vi "ROSTerminal.vi"() -> ()   [LabVIEW 2015]
doc: "Provides a space to debug any errors in code by:\n-allowing for testing connection to master\n-showing open nodes\n-linking to a website for viewing what is passed back and forth on a topic\n-linking to a website for the master to view what is passed back and forth\n-showing open logs\n-providing IP for you and Master"
uses:
  _ROSDefinition.vi
  vi.lib/Platform/browser.llb/Open URL in Default Browser (string).vi
  SubVIs/_ROSDirection.ctl
  SubVIs/_ROSControl.ctl
panel:
  in  "Change IP":bool
  in  "CloseServer":bool
  out "Queue Contents":string[](array[string])
  in  "ClearAllLogs":bool
  in  "CloseServers":bool
  in  "LabVIEW Servers":i32(listbox)
  in  "ClearOldLogs":bool
  in  "Web Logs":i32(listbox)
  in  "OpenNodes":bool
  in  "MasterWeb":bool
  in  "MyWeb":bool
  in  "UDP":bool
  out "My IP":string="http://192.168.1.8"
  in  "Done":bool
  out "Live":bool
  in  "Test":bool
  in  "Current Master":string="192.168.1.110:11311"
  # "Displays queue size and contents. Double click for\nmore information on a particular server."
  # "Show commands sent over TCP. \nDouble click to open a web page."
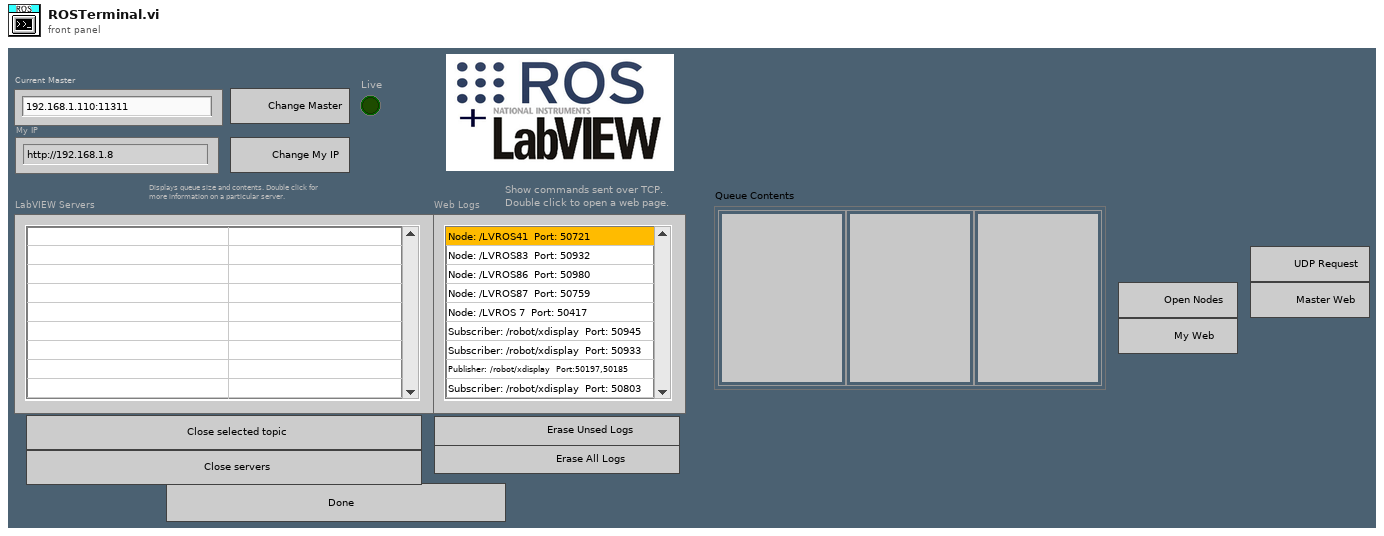
[diagram p1: front panel]
types:
  T1 = enum8{"Enabled", "Disabled", "Disabled and Grayed Out"}
  T2 = typedef "_ROSControl.ctl" = cluster{"topic port":u16, "Node":string, "topic":string, "type":string, "node port":u16, "error ":errorcluster, "Direction":T3, "Update (ms)":u16, "FIFO size":u16}
  T3 = typedef "_ROSDirection.ctl" = enum16{"Node", "Publisher", "Subscriber", "ServiceClient", "ServiceProvider"}
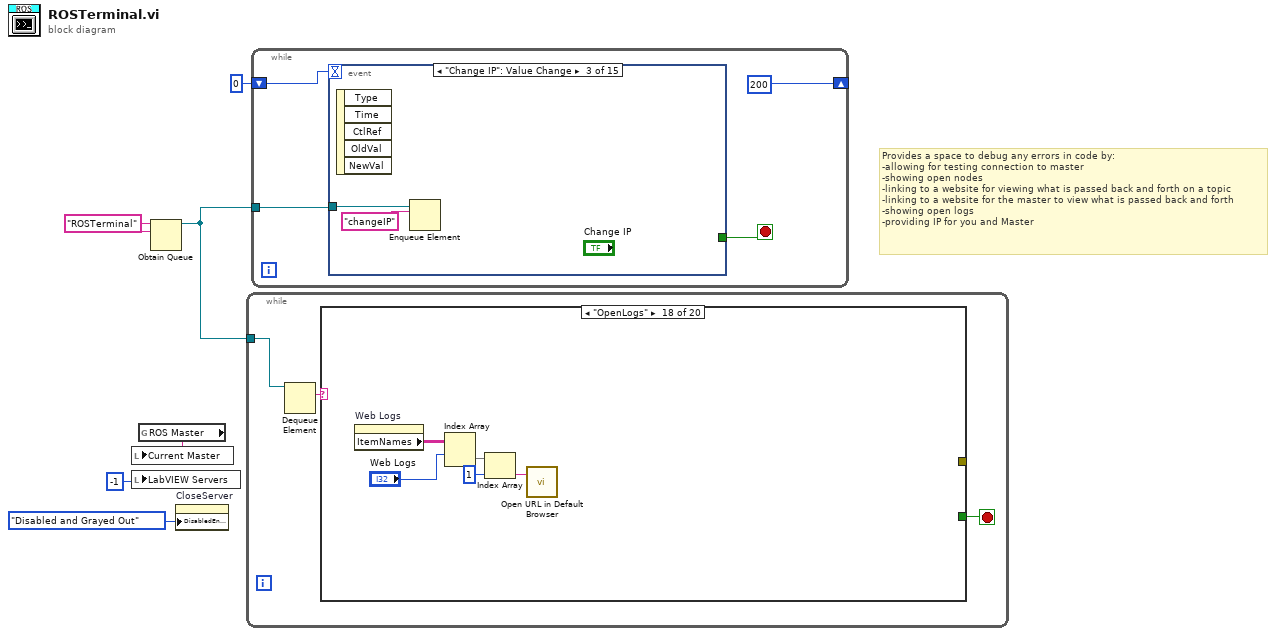
[diagram p0: block diagram]
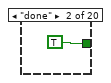
[diagram p3: hidden frame]
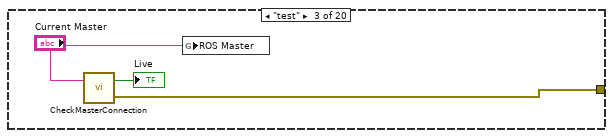
[diagram p4: hidden frame]
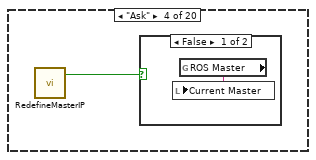
[diagram p5: hidden frame]
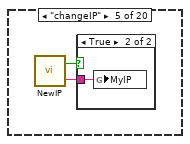
[diagram p7: hidden frame]
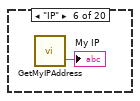
[diagram p9: hidden frame]
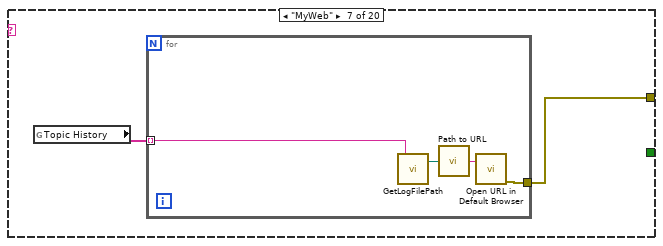
[diagram p10: hidden frame]
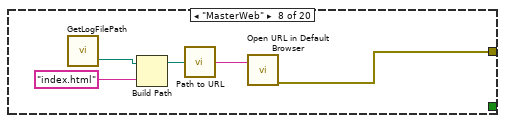
[diagram p11: hidden frame]
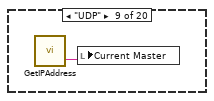
[diagram p12: hidden frame]
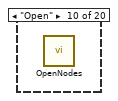
[diagram p13: hidden frame]
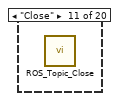
[diagram p14: hidden frame]
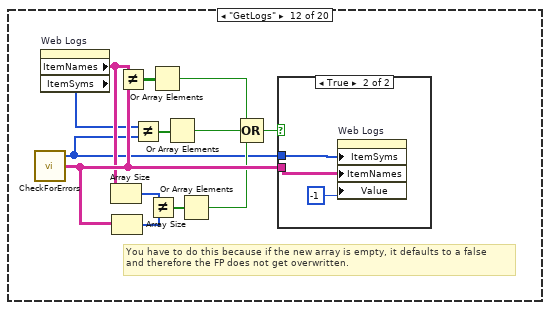
[diagram p15: hidden frame]
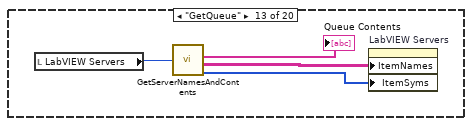
[diagram p17: hidden frame]
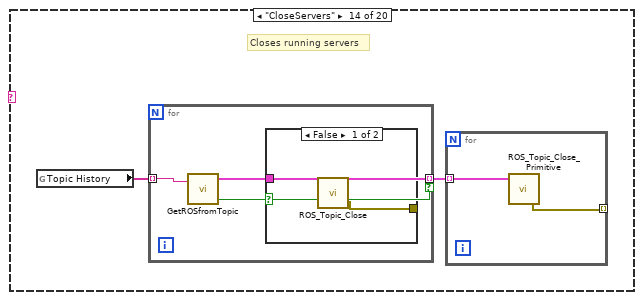
[diagram p18: hidden frame]
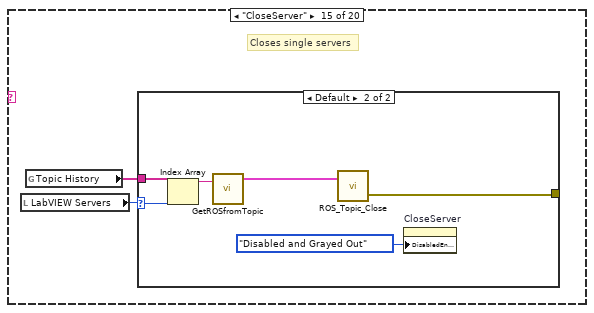
[diagram p20: hidden frame]
diagram:
  w5 = "ROSTerminal" ("name (unnamed)")
  # "Provides a space to debug any errors in code by:\n-allowing for testing connection to master\n-showing open nodes\n-linking to a website for viewing what is passed back and forth on a topic\n-linking to a website for the master to view what is passed back and forth\n-showing open logs\n-providing IP for you and Master"
  n1 = local write "LabVIEW Servers"(-1 ("Nodes")) -> ()
  n2 = global read "_ROSDefinition.vi" "ROS Master"() -> (w6:string)
  n3 = local write "Current Master"(w6) -> ()
  n4 = Obtain Queue(name (unnamed)=w5, element data type=w5) -> (queue out=w3:refnum<queue>)  [unwired: 3 in, 2 out]
  n5 = property on="CloseServer" class="Bool"("DisabledEnum"=T1."Disabled and Grayed Out" ("Disabled")) -> ()  [unwired: 2 in, 2 out]
  n6 = while {
    tunnel: w3 -> [w9]
    stop <- w7 stop-if-true
    n7 = Dequeue Element(queue=w9) -> (element=w8:string)  [unwired: 2 in, 3 out]
    n8 = case shown="\"OpenLogs\"" w8 {
      tunnel: [_ TRUE _ _ _ _ _ _ _ _ _ _ _ _ _ _ _ _ _ _] -> w7
      tunnel: [_ _ w11 _ _ _ w21 w26 _ _ _ _ _ _ _ w70 _ _ _ _] -> _
      frame Default {
      }
      frame "done" {
      }
      frame "test" {
        n9 = call "CheckMasterConnection.vi"("Master IP"="Current Master") -> ("error out"=w11:errorcluster, "Master There?"=→"Live":bool)  [unwired: 1 in]
        n10 = global write "_ROSDefinition.vi" "ROS Master"("Current Master") -> ()
      }
      frame "Ask" {
        n11 = call "RedefineMasterIP.vi"() -> ("Abort?"=w14:bool)  [unwired: 2 in]
        n12 = case shown="False" w14 {
          frame False {
            n13 = global read "_ROSDefinition.vi" "ROS Master"() -> (w15:string)
            n14 = local write "Current Master"(w15) -> ()
          }
          frame True {
          }
        }
      }
      frame "changeIP" {
        n15 = call "NewIP.vi"() -> ("New IP"=w16:string, "New IP?"=w17:bool)  [unwired: 2 in]
        n16 = case shown="True" w17 {
          tunnel: w16 -> [_ w18]
          frame False {
          }
          frame True {
            n17 = global write "_ROSDefinition.vi" "MyIP"(w18) -> ()
          }
        }
      }
      frame "IP" {
        n18 = call "GetMyIPAddress.vi"() -> ("URI"=→"My IP":string)  [unwired: 2 in, 1 out]
      }
      frame "MyWeb" {
        n19 = global read "_ROSDefinition.vi" "Topic History"() -> (w20:string[])
        n20 = for {
          tunnel: [w24] -> w21
          tunnel: w20 -> [w22] mode=indexing
          n21 = call "GetLogFilePath.vi"("Server name"=w22) -> ("LogPath"=w23:path)  [unwired: 1 in, 1 out]
          n22 = call "Path to URL.vi"("path"=w23) -> ("url"=w25:string)
          n23 = call-poly "Open URL in Default Browser.vi"("URL"=w25) -> ("error out"=w24:errorcluster)  [unwired: 5 in, 1 out]
        }
      }
      frame "MasterWeb" {
        n24 = call "GetLogFilePath.vi"() -> ("LogFolder"=w29:path)  [unwired: 2 in, 1 out]
        n25 = Build Path(base path=w29, name or relative path="index.html") -> (appended path=w27:path)
        n26 = call "Path to URL.vi"("path"=w27) -> ("url"=w30:string)
        n27 = call-poly "Open URL in Default Browser.vi"("URL"=w30) -> ("error out"=w26:errorcluster)  [unwired: 5 in, 1 out]
      }
      frame "UDP" {
        n28 = call "GetIPAddress.vi"() -> ("data out"=w31:string)  [unwired: 3 in]
        n29 = local write "Current Master"(w31) -> ()
      }
      frame "Open" {
        n30 = call "OpenNodes.vi"() -> ()  [unwired: 2 in]
      }
      frame "Close" {
        n31 = call "ROS_Topic_Close.vi"() -> ()  [unwired: 4 in, 1 out]
      }
      frame "GetLogs" {
        # "You have to do this because if the new array is empty, it defaults to a false\nand therefore the FP does not get overwritten."
        n32 = call "CheckForErrors.vi"() -> ("Symbols"=w33:i32[], "Logs"=w43:string[][])  [unwired: 2 in, 1 out]
        n33 = property on="Web Logs" class="MCListbox (strict)"() -> ("ItemNames"=w42:string[][], "ItemSyms"=w34:i32[])  [unwired: 2 in, 2 out]
        n34 = Array Size(array=w42) -> (size(s)=w41:i32[])
        n35 = Array Size(array=w43) -> (size(s)=w40:i32[])
        n36 = Not Equal?(x=w42, y=w43) -> (x != y?=w44:bool[][])
        n37 = Not Equal?(x=w34, y=w33) -> (x != y?=w35:bool[])
        n38 = Not Equal?(x=w41, y=w40) -> (x != y?=w39:bool[])
        n39 = Or Array Elements(Boolean array=w44) -> (logical OR=w38:bool)
        n40 = Or Array Elements(Boolean array=w35) -> (logical OR=w32:bool)
        n41 = Or Array Elements(Boolean array=w39) -> (logical OR=w37:bool)
        n42 = Compound Arithmetic op=OR(w38, w32, w37) -> (w36:bool)
        n43 = case shown="True" w36 {
          tunnel: w33 -> [_ w46]
          tunnel: w43 -> [_ w45]
          frame False {
          }
          frame True {
            n44 = property on="Web Logs" class="MCListbox (strict)"("ItemSyms"=w46, "ItemNames"=w45, "Value"=-1 ("Listbox")) -> ()  [unwired: 2 in, 2 out]
          }
        }
      }
      frame "GetQueue" {
        n45 = local read "LabVIEW Servers"() -> (w49:i32)
        n46 = call "GetServerNamesAndContents.vi"("Desired Server"=w49) -> ("Queue Contents"=→"Queue Contents":string[], "Nice Names"=w48:string[][], "Symbols"=w51:i32[])  [unwired: 1 out]
        n47 = property on="LabVIEW Servers" class="MCListbox (strict)"("ItemNames"=w48, "ItemSyms"=w51) -> ()  [unwired: 2 in, 2 out]
      }
      frame "CloseServers" {
        # "Closes running servers"
        n48 = global read "_ROSDefinition.vi" "Topic History"() -> (w53:string[])
        n49 = for {
          tunnel: w53 -> [w58] mode=indexing
          tunnel: [w57] -> w52 mode=indexing if=w56
          n50 = call "GetROSfromTopic.vi"("Topic"=w58) -> ("ROS"=w57:T2, "Node?"=w56:bool)  [unwired: 1 in, 1 out]
          n51 = case shown="False" w56 {
            tunnel: w57 -> [w60 _]
            tunnel: [w59 _] -> _
            frame False {
              n52 = call "ROS_Topic_Close.vi"("ROS in"=w60) -> ("error out"=w59:errorcluster)  [unwired: 3 in]
            }
            frame True {
            }
          }
        }
        n53 = for {
          tunnel: w52 -> [w55] mode=indexing
          tunnel: [w54] -> _ mode=indexing
          n54 = call "ROS_Topic_Close_Primitive.vi"("ROS in"=w55) -> ("error out"=w54:errorcluster)  [unwired: 2 in]
        }
      }
      frame "CloseServer" {
        # "Closes single servers"
        n55 = local read "LabVIEW Servers"() -> (w61:i32)
        n56 = global read "_ROSDefinition.vi" "Topic History"() -> (w62:string[])
        n57 = case shown="Default" w61 {
          selector: w61 -> [_ w67]
          tunnel: w62 -> [_ w66]
          tunnel: [_ w63] -> _
          frame -1 {
          }
          frame Default {
            n58 = Index Array(array=w66, index=w67) -> (element=w65:string)
            n59 = call "GetROSfromTopic.vi"("Topic"=w65) -> ("ROS"=w68:T2)  [unwired: 1 in, 2 out]
            n60 = call "ROS_Topic_Close.vi"("ROS in"=w68) -> ("error out"=w63:errorcluster)  [unwired: 3 in]
            n61 = property on="CloseServer" class="Bool"("DisabledEnum"=T1."Disabled and Grayed Out" ("Disabled")) -> ()  [unwired: 2 in, 2 out]
          }
        }
      }
      frame "OpenServer" {
        # "Opens a server"
        n62 = global read "_ROSDefinition.vi" "Topic History"() -> (w75:string[])
        n63 = Index Array(array=w75, index="LabVIEW Servers") -> (element=w73:string)
        n64 = call "GetROSfromTopic.vi"("Topic"=w73) -> ("ROS"=w71:T2)  [unwired: 1 in, 2 out]
        n65 = call "ROSToQueue.vi"("ROS"=w71) -> ("error out"=w69:errorcluster, "queue"=w72:refnum<queue>)  [unwired: 3 in]
        n66 = Enqueue Element(queue=w72, element="show", error in (no error)=w69) -> (error out=w70:errorcluster)  [unwired: 1 in, 2 out]
      }
      frame "OpenLogVI" {
        n67 = property on="Web Logs" class="MCListbox (strict)"() -> ("ItemNames"=w81:string[][], "Value"=w82:i32)  [unwired: 2 in, 2 out]
        n68 = Index Array(array=w81, index (row)=w82, index (col)=3 ("disabled index (col)")) -> (element=w86:string)
        n69 = Match Pattern(string=w86, regular expression="(") -> (before substring=w78:string, after substring=w87:string)  [unwired: 1 in, 2 out]
        n70 = Match Pattern(string=w87, regular expression=")") -> (before substring=w80:string, after substring=w89:string)  [unwired: 1 in, 2 out]
        n71 = call "Trim Whitespace.vi"("string"=w78) -> ("trimmed string"=w77:string)  [unwired: 1 in]
        n72 = call "Trim Whitespace.vi"("string"=w80) -> ("trimmed string"=w79:string)  [unwired: 1 in]
        n73 = case shown="\"Publisher\"" w89 {
          tunnel: T2 {"topic port"=0, "Node"="/fred", "topic"="/robot/head/command_head_nod", "type"="std_msgs/Bool", "node port"=59377, "error "={"status"=FALSE, "code"=0, "source"=""}, "Direction"=enum."Publisher", "Update (ms)"=1, "FIFO size"=1} ("ROS") -> [_ w98 w107 w116]
          tunnel: w77 -> [_ w92 w102 w111]
          tunnel: w79 -> [_ w91 w101 w110]
          tunnel: [_ w90 w99 w108] -> _
          frame Default {
          }
          frame "Publisher" {
            n74 = Bundle By Name(cluster=w98, "Node"=w91, "topic"=w92, "Direction"=_ROSDirection."Publisher") -> (w97:T2)
            n75 = call "ROSToQueue.vi"("ROS"=w97, "Name"=enum16{"topic", "node"}."topic") -> ("queue"=w95:refnum<queue>)  [unwired: 2 in, 1 out]
            n76 = Enqueue Element(queue=w95, element="show") -> (error out=w90:errorcluster)  [unwired: 2 in, 2 out]
          }
          frame "Subscriber" {
            n77 = Bundle By Name(cluster=w107, "Node"=w101, "topic"=w102, "Direction"=_ROSDirection."Subscriber") -> (w106:T2)
            n78 = call "ROSToQueue.vi"("ROS"=w106, "Name"=enum16{"topic", "node"}."topic") -> ("queue"=w104:refnum<queue>)  [unwired: 2 in, 1 out]
            n79 = Enqueue Element(queue=w104, element="show") -> (error out=w99:errorcluster)  [unwired: 2 in, 2 out]
          }
          frame "Node" {
            n80 = Bundle By Name(cluster=w116, "Node"=w110, "topic"=w111, "Direction"=_ROSDirection."Node") -> (w115:T2)
            n81 = call "ROSToQueue.vi"("ROS"=w115, "Name"=enum16{"topic", "node"}."node") -> ("queue"=w113:refnum<queue>)  [unwired: 2 in, 1 out]
            n82 = Enqueue Element(queue=w113, element="show") -> (error out=w108:errorcluster)  [unwired: 2 in, 2 out]
          }
        }
      }
      frame "OpenLogs" {
        n83 = property on="Web Logs" class="MCListbox (strict)"() -> ("ItemNames"=w121:string[][])  [unwired: 2 in, 2 out]
        n84 = Index Array(array=w121, index (row)="Web Logs") -> (element=w120:string[])  [unwired: 1 in]
        n85 = Index Array(array=w120, index=1) -> (element=w117:string)
        n86 = call-poly "Open URL in Default Browser.vi"("URL"=w117) -> ()  [unwired: 5 in, 2 out]
      }
      frame "EraseLogs" {
        n87 = call "CheckForErrors.vi"() -> ("Symbols"=w123:i32[], "Paths"=w122:path[])  [unwired: 2 in, 1 out]
        n88 = for {
          tunnel: w123 -> [w125] mode=indexing
          tunnel: w122 -> [w124] mode=indexing
          n89 = case shown="0" w125 {
            tunnel: [w127 _] -> _
            tunnel: w124 -> [w126 _]
            frame 0 {
              n90 = Delete(path (use dialog)=w126) -> (error out=w127:errorcluster)  [unwired: 4 in, 2 out]
            }
            frame Default {
            }
          }
        }
      }
      frame "EraseAll" {
        n91 = call "CheckForErrors.vi"() -> ("Paths"=w128:path[])  [unwired: 2 in, 2 out]
        n92 = for {
          tunnel: w128 -> [w130] mode=indexing
          tunnel: [w129] -> _ mode=indexing
          n93 = Delete(path (use dialog)=w130) -> (error out=w129:errorcluster)  [unwired: 4 in, 2 out]
        }
      }
    }
  }
  n94 = while {
    tunnel: w3 -> [w134]
    shift-right: [200 ("timeout in ms (-1)")] -> _
    shift-left: 0 ("timeout in ms (-1)") -> [w131]
    stop <- w133 stop-if-true
    n95 = event shown="[2] \"Change IP\": Value Change" {
      selector: _ -> [_ _ _ _ _ _ _ _ _ _ _ _ _ _ _]
      dyn-events: _ -> [_ _ _ _ _ _ _ _ _ _ _ _ _ _ _]
      timeout: w131 -> [_ _ _ _ _ _ _ _ _ _ _ _ _ _ _]
      tunnel: w134 -> [w136 w144 w146 w148 w150 w152 _ w155 w157 w159 w163 w167 w169 w171 w174]
      tunnel: [_ _ _ _ _ _ _ _ _ _ _ _ _ _ "Done"] -> w133
      event Timeout {
        n96 = event-data() -> ()  [unwired: 1 in, 1 out]
        n97 = Get Queue Status(queue=w136) -> (# elements in queue=w135:i32)  [unwired: 2 in, 7 out]
        n98 = case shown="0" w135 {
          tunnel: string[] ["IP", "GetLogs", "test", "GetQueue"] -> [_ w139]
          tunnel: w136 -> [_ w138]
          frame Default {
          }
          frame 0 {
            n99 = for {
              shift-right: [w142] -> _
              shift-left: w138 -> [w141]
              tunnel: w139 -> [w140] mode=indexing
              n100 = Enqueue Element(queue=w141, element=w140) -> (queue out=w142:refnum<queue>)  [unwired: 2 in, 2 out]
            }
          }
        }
      }
      event "Test", "Current Master": Value Change {
        n101 = event-data() -> ()  [unwired: 1 in, 1 out]
        n102 = Enqueue Element(queue=w144, element="Ask") -> ()  [unwired: 2 in, 3 out]
      }
      event "Change IP": Value Change {
        n103 = event-data() -> ()  [unwired: 1 in, 5 out]
        n104 = Enqueue Element(queue=w146, element="changeIP") -> ()  [unwired: 2 in, 3 out]
      }
      event "MyWeb": Value Change {
        n105 = event-data() -> ()  [unwired: 1 in, 1 out]
        n106 = Enqueue Element(queue=w148, element="MyWeb") -> ()  [unwired: 2 in, 3 out]
      }
      event "UDP": Value Change {
        n107 = event-data() -> ()  [unwired: 1 in, 1 out]
        n108 = Enqueue Element(queue=w150, element="UDP") -> ()  [unwired: 2 in, 3 out]
      }
      event "LabVIEW Servers": Double Click {
        n109 = event-data() -> ()  [unwired: 1 in, 1 out]
        n110 = Enqueue Element(queue=w152, element="OpenServer") -> ()  [unwired: 2 in, 3 out]
      }
      event "LabVIEW Servers": Mouse Up {
        n111 = event-data() -> ()  [unwired: 1 in, 1 out]
        n112 = property on="CloseServer" class="Bool"("DisabledEnum"=T1."Enabled" ("Disabled")) -> ()  [unwired: 2 in, 2 out]
      }
      event "Web Logs": Double Click {
        n113 = event-data() -> ()  [unwired: 1 in, 1 out]
        n114 = Enqueue Element(queue=w155, element="OpenLogs") -> ()  [unwired: 2 in, 3 out]
      }
      event "CloseServers": Value Change {
        n115 = event-data() -> ()  [unwired: 1 in, 5 out]
        n116 = Enqueue Element(queue=w157, element="CloseServers") -> ()  [unwired: 2 in, 3 out]
      }
      event "CloseServer": Value Change {
        n117 = event-data() -> ()  [unwired: 1 in, 5 out]
        n118 = Enqueue Element(queue=w159, element="CloseServer") -> ()  [unwired: 2 in, 3 out]
      }
      event "ClearOldLogs": Value Change {
        n119 = event-data() -> ()  [unwired: 1 in, 5 out]
        n120 = Enqueue Element(queue=w163, element="EraseLogs") -> (queue out=w161:refnum<queue>)  [unwired: 2 in, 2 out]
        n121 = Enqueue Element(queue=w161, element="GetLogs") -> ()  [unwired: 2 in, 3 out]
      }
      event "ClearAllLogs": Value Change {
        n122 = event-data() -> ()  [unwired: 1 in, 5 out]
        n123 = Enqueue Element(queue=w167, element="EraseAll") -> (queue out=w165:refnum<queue>)  [unwired: 2 in, 2 out]
        n124 = Enqueue Element(queue=w165, element="GetLogs") -> ()  [unwired: 2 in, 3 out]
      }
      event "OpenNodes": Value Change {
        n125 = event-data() -> ()  [unwired: 1 in, 1 out]
        n126 = Enqueue Element(queue=w169, element="Open") -> ()  [unwired: 2 in, 3 out]
      }
      event "MasterWeb": Value Change {
        n127 = event-data() -> ()  [unwired: 1 in, 1 out]
        n128 = Enqueue Element(queue=w171, element="MasterWeb") -> ()  [unwired: 2 in, 3 out]
      }
      event "Done": Value Change {
        n129 = event-data() -> ()  [unwired: 1 in, 1 out]
        n130 = Enqueue Element(queue=w174, element="done") -> ()  [unwired: 2 in, 3 out]
      }
    }
  }
